vi "DMM Configuration - Convert DMM Range Strings into EU.vi"(8 "error in (no error)":errorcluster, 9 "DMM Range ComboBox Strings":string[](array[string]), 10 "Dmm Range Index In":u16) -> (0 "error out":errorcluster, 2 "DMM Range [EU]":dbl)   [LabVIEW 2015, in "DMM-SWITCH-ScanList System Explorer.lvlib"]
doc: "Gets the DMM Range ComboBox Strings and calculates the corresponding range"
uses:
  DMM-SWITCH-ScanList System Explorer.lvlib
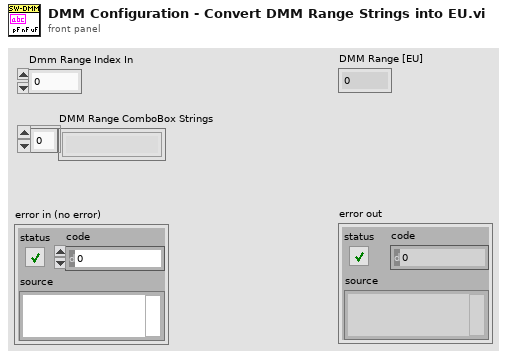
[diagram p1: front panel]
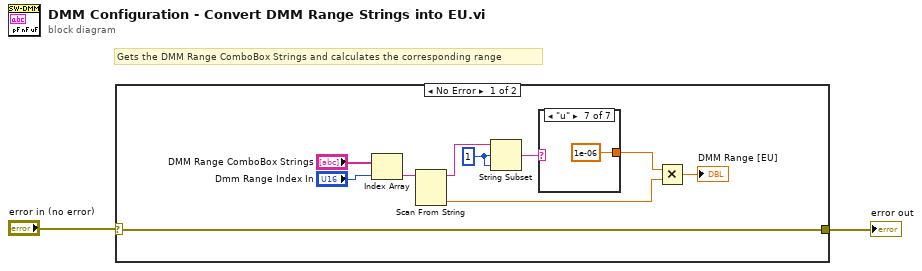
[diagram p0: block diagram]
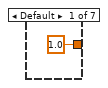
[diagram p2: hidden frame]
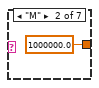
[diagram p3: hidden frame]
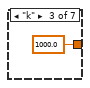
[diagram p4: hidden frame]
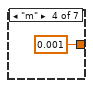
[diagram p5: hidden frame]
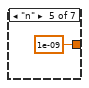
[diagram p6: hidden frame]
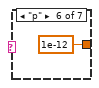
[diagram p7: hidden frame]
diagram:
  # "Gets the DMM Range ComboBox Strings and calculates the corresponding range"
  n1 = case shown="No Error" "error in (no error)" {
    selector: "error in (no error)" -> [w3 w20]
    tunnel: [w3 w20] -> w1
    frame No Error {
      w6 = 1 ("offset (0)")
      n2 = Index Array(array="DMM Range ComboBox Strings", index="Dmm Range Index In") -> (element=w8:string)
      n3 = Scan From String(input string=w8) -> (remaining string=w7:string, output 1=w5:dbl)  [unwired: 4 in, 2 out]
      n4 = String Subset(string=w7, offset (0)=w6, length (rest)=w6) -> (substring=w9:string)
      n5 = case shown="\"u\"" w9 {
        tunnel: [1.0 1000000.0 1000.0 0.001 1e-09 1e-12 1e-06] -> w10
        frame Default {
        }
        frame "M" {
        }
        frame "k" {
        }
        frame "m" {
        }
        frame "n" {
        }
        frame "p" {
        }
        frame "u" {
        }
      }
      n6 = Multiply(x=w10, y=w5) -> (x*y=→"DMM Range [EU]":dbl)
    }
    frame Error {
    }
  }
  "error out" <- w1
